vi "Run Error Handler in the Background.vi"(7 "node-ID":u8, 8 "error in (no error)":errorcluster, 11 "interface object in":refnum<k20>) -> (0 "error out":errorcluster, 3 "interface object out":refnum<k20>)   [LabVIEW 2016]
uses:
  <vilib>/CANopenLib/CANOPEN.llb/CANopen Emergency Create.vi
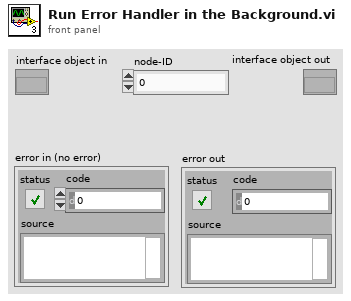
[diagram p1: front panel]
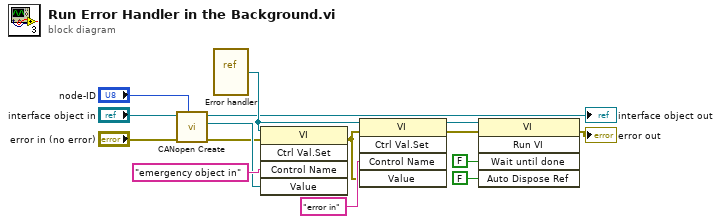
[diagram p0: block diagram]
diagram:
  n1 = call-poly <vilib>:"CANopen Create.vi"("node-ID"="node-ID", "error in (no error)"="error in (no error)", "interface object in"="interface object in") -> ("error out"=w3:errorcluster, "emergency object out"=w6:refnum<k20>, "interface object out"=→"interface object out":refnum<k20>)  [unwired: 6 in]
  n2 = vi-ref "Error handler.vi"() -> (w8:refnum<vi>)
  n3 = invoke class="VI" method="Ctrl Val.Set"(reference=w8, error in=w3, "Control Name"="emergency object in", "Value"=w6) -> (error out=w11:errorcluster)  [unwired: 1 in, 4 out]
  n4 = invoke class="VI" method="Ctrl Val.Set"(reference=w8, error in=w11, "Control Name"="error in", "Value"=w11) -> (reference out=w9:refnum<vi>, error out=w10:errorcluster)  [unwired: 1 in, 3 out]
  n5 = invoke class="VI" method="Run VI"(reference=w9, error in=w10, "Wait until done"=FALSE ("Wait Until Done"), "Auto Dispose Ref"=FALSE ("Auto Dispose Reference")) -> (error out=→"error out":errorcluster)  [unwired: 1 in, 4 out]
